vi "Basic UART loop.vi"() -> ()   [LabVIEW 2017]
uses:
  <vilib>/myRIO/Instrument Drivers/Onboard IO/UART/typedef/VISA Configuration.ctl
  <vilib>/myRIO/Instrument Drivers/Onboard IO/UART/UART.lvlib
panel:
  out "error?":bool
  in  "stop":bool
  out "read buffer":string
  in  "Read mode":enum16{"Read all", "Get latest value"}(ring)=enum."Get latest value"
  in  "VISA resource name in":refnum<visa-resource-name>="ASRL1::INSTR"
  out "Loop num":i32
  out "timeout (10sec)":u32
  in  "input cluster":T1={"baud rate (9600)"=115200, "data bits (8)"=8, "parity (0:none)"=enum."None", "stop bits (10: 1 bit)"=10, "flow control (0:none)"=0, "termination char\n(0xA = '\\n' = LF) "=10, "Enable Termination\nChar (T)"=TRUE, "timeout (10sec)"=1000} {"termination char\n(0xA = '\\n' = LF)" format="%.0x"; "flow control (0:none)" items=["None", "XON/XOFF", "RTS/CTS", "XON/XOFF & RTS/CTS", "DTR/DSR", "XON/XOFF & DTR/DSR"]; "stop bits (10: 1 bit)" items=["1.0"=10, "1.5"=15, "2.0"=20]; "data bits (8)" min=5 max=8 step=1}
  out "error out":errorcluster
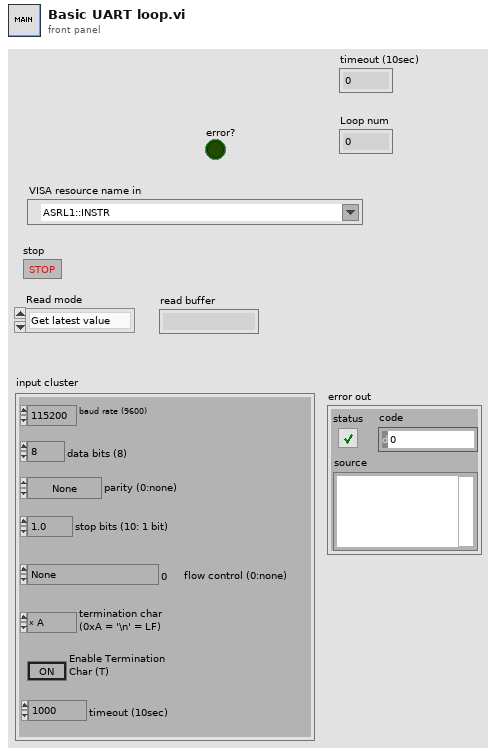
[diagram p1: front panel]
types:
  T1 = typedef "UART.lvlib/VISA Configuration.ctl" = cluster{"baud rate (9600)":u32, "data bits (8)":u16, "parity (0:none)":enum16{"None", "Odd", "Even", "Mark", "Space"}, "stop bits (10: 1 bit)":u16, "flow control (0:none)":u16, "termination char\n(0xA = '\\n' = LF) ":u8, "Enable Termination\nChar (T)":bool, "timeout (10sec)":u32}
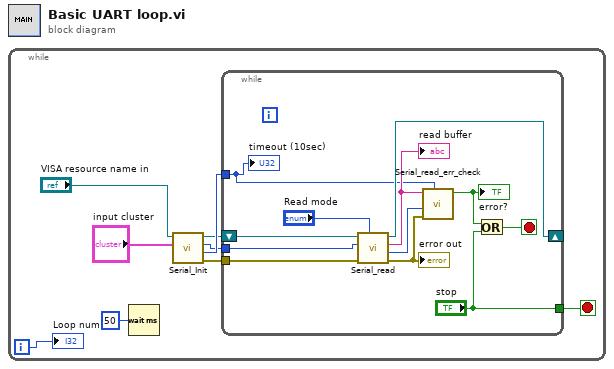
[diagram p0: block diagram]
diagram:
  n1 = while {
    i -> [w1]
    stop <- w3 stop-if-true
    n2 = Wait (ms)(milliseconds to wait=u32 50) -> ()  [unwired: 1 out]
    n3 = call "Serial_Init.vi"("input cluster"="input cluster", "VISA Refnum in"="VISA resource name in") -> ("error out"=w8:errorcluster, "timeout (10sec)"=w7:u32, "Bytes at Port"=w6:u32, "VISA Refnum out"=w5:refnum<visa-resource-name>)  [unwired: 6 in]
    n4 = while {
      tunnel: w8 -> [w20]
      tunnel: w7 -> [w13]
      tunnel: w6 -> [w19]
      shift-right: [w17] -> _
      shift-left: w5 -> [w18]
      tunnel: ["stop"] -> w3
      stop <- w11 stop-if-true
      n5 = call "Serial_read.vi"("Read mode"="Read mode", "error in (no error)"=w20, "Bytes at Port"=w19, "VISA Refnum in"=w18) -> ("error out"=w15:errorcluster, "dt"=w14:u32, "read buffer"=w16:string, "VISA resource name out"=w17:refnum<visa-resource-name>)  [unwired: 4 in]
      "error out" <- w15
      "read buffer" <- w16
      n6 = call "Serial_read_err_check.vi"("timeout"=w13, "error in (no error)"=w15, "dt"=w14, "read buffer"=w16) -> ("error?"=w10:bool)  [unwired: 7 in]
      "error?" <- w10
      n7 = Or(x=w10, y="stop") -> (x .or. y?=w11:bool)
      "timeout (10sec)" <- w13
    }
    "Loop num" <- w1
  }
